vi "主程序.vi"() -> ()   [LabVIEW 2010]
panel:
  out "test_k":dbl
  in  "test_x1":dbl
  in  "test_x2":dbl
  in  "test_y1":dbl
  in  "test_y2":dbl
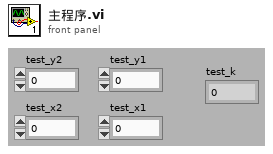
[diagram p1: front panel]
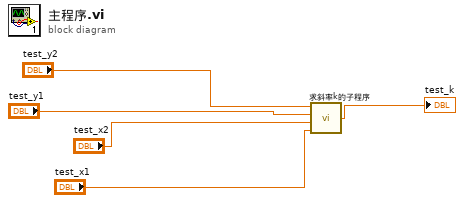
[diagram p0: block diagram]
diagram:
  n1 = call "求斜率k的子程序.vi"("x1"="test_x1", "x2"="test_x2", "y1"="test_y1", "y2"="test_y2") -> ("k"=→"test_k":dbl)
